vi "TextEditTable.vi"() -> ()   [LabVIEW 2018]
doc: "Handle edits in a text table, limited to column 0\nClick mouse to start edit, Enter to finish edit.\n\n* React to Enter key to complete edit\n* Grab cell one row above the current edit cell (because the table has already responded to the Enter key by moving the current edit cell down by one)\n* Limit edits to only certain rows/cols or cells by changing focus to a dummy offscreen control. (Note: if this dummy control is \"hidden\", this trick won't work).\n* I used a sequence structure to ensure that data gets pulled from table cell _after_ edit has completed (otherwise, it would pull the data before the edit was done)\n*escape key automatically works as it should: it gives up focus and returns the edit cell contents to the string that was there before the edit.\n\nCopyright © 2011 Epimedia, Inc. All Rights Reserved.\n\nThe Epimedia Application Library is Copyright © 2009-2011 Epimedia, Inc. \nAll Rights Reserved. Used under license."
uses:
  <vilib>/Utility/miscctls.llb/LVRowAndColumnTypeDef.ctl
  <vilib>/event_ctls.llb/lveventtype.ctl
  <vilib>/event_ctls.llb/eventvkey.ctl
panel:
  out "SavedDataAfterEdit":string
  in  "DummyButton":bool
  out "Mods":cluster{"Num Pad":bool, "Menu Key":bool}
  out "ScanCode":i16
  out "VKey":T1
  out "Char":i16
  out "Type":T2
  in  "stop":bool
  out "CellValBeforeEdit":string
  out "Active Cell:Active Cell":T3
  in  "Worker Status":string[][](table)
  # "Copyright © 2011 Epimedia, Inc. All Rights Reserved.\n\nThe Epimedia Application Library is Copyright © 2009-2011 Epimedia, Inc. \nAll Rights Reserved. Used under license."
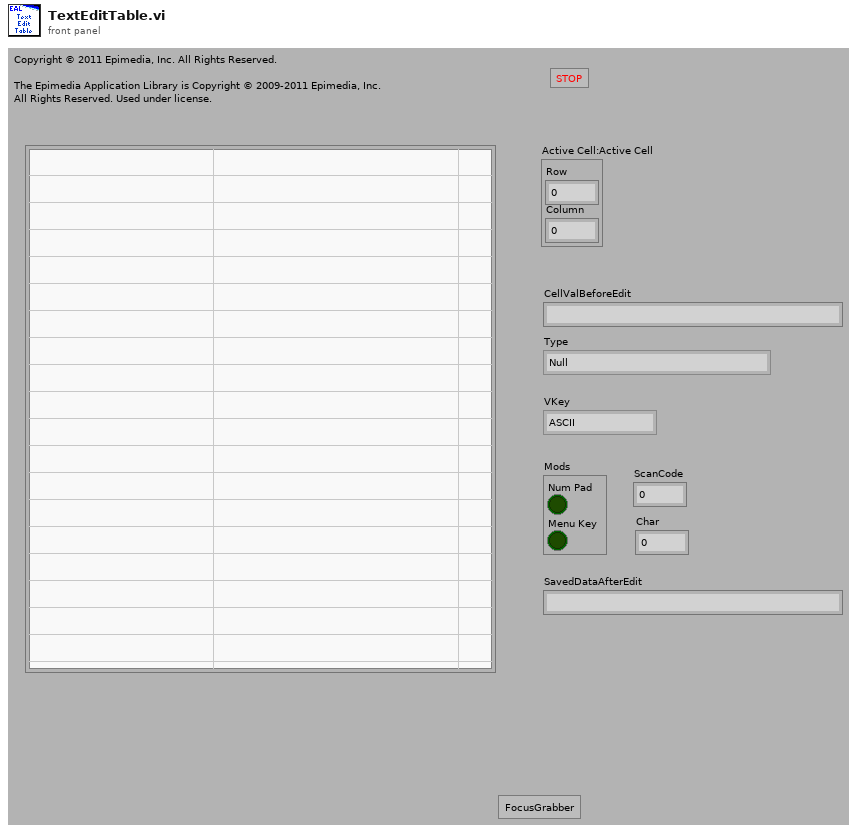
[diagram p1: front panel]
types:
  T1 = typedef "eventvkey.ctl" = enum16{"ASCII", "Enter", "Return", "Shift", "Ctrl", "Alt", "Cmd", "Opt", "Caps", "NumLock", "Clear", "Break", "Up", "Down", "Left", "Right", "Insert", "Delete", "Home", "End", "PageUp", "PageDown", "Escape", "Help", "Pause", "ScrollLock", "F1", "F2", "F3", "F4", "F5", "F6", "F7", "F8", "F9", "F10", "F11", "F12", "F13", "F14", "F15", "F16", "F17", "F18", "F19", "F20", "F21", "F22", "F23", "F24", "Play", "VolumeUp", "VolumeDown", "Mute", "Two Byte Char"}
  T2 = typedef "lveventtype.ctl" = enum32{"Null", "Timeout", "Annotation Menu Selection", "Annotation Menu Selection?", "App Instance Close", "App Instance Close?", "Autoscale Range Change", "Bookmark Info Change", "Cell Edit", "Cell Edit?", "Cursor Grab", "Cursor Grab?", "Cursor Menu Selection", "Cursor Menu Selection?", "Cursor Move", "Cursor Release", "Data Change", "Direction Change", "Display State Change", "Drag Ended", "Drag Enter", "Drag Leave", "Drag Over", "Drag Source Update", "Drag Starting", "Drag Starting?", "Drop", "Exec State Change", "Key Down", "Key Down?", "Key Repeat", "Key Repeat?", "Key Up", "Listbox Double Click", "Menu Activation?", "Menu Selection (App)", "Menu Selection? (App)", "Menu Selection (User)", "Mouse Down", "Mouse Down?", "Mouse Enter", "Mouse Leave", "Mouse Move", "Mouse Up", "Mouse Wheel", "NI Security User Change (App)", "Pane Size", "Panel Close", "Panel Close?", "Panel Resize", "Plot Attribute Change", "Scale Range Change", "Shortcut Menu Activation?", "Shortcut Menu Selection (App)", "Shortcut Menu Selection? (App)", "Shortcut Menu Selection (User)", "Tree Double Click", "Tree Drag", "Tree Drag?", "Tree Drop", "Tree Drop?", "Tree Item Close", "Tree Item Close?", "Tree Item Open", "Tree Item Open?", "User Event", "Value Change"}
  T3 = typedef "LVRowAndColumnTypeDef.ctl" = cluster{"Row":i32, "Column":i32}
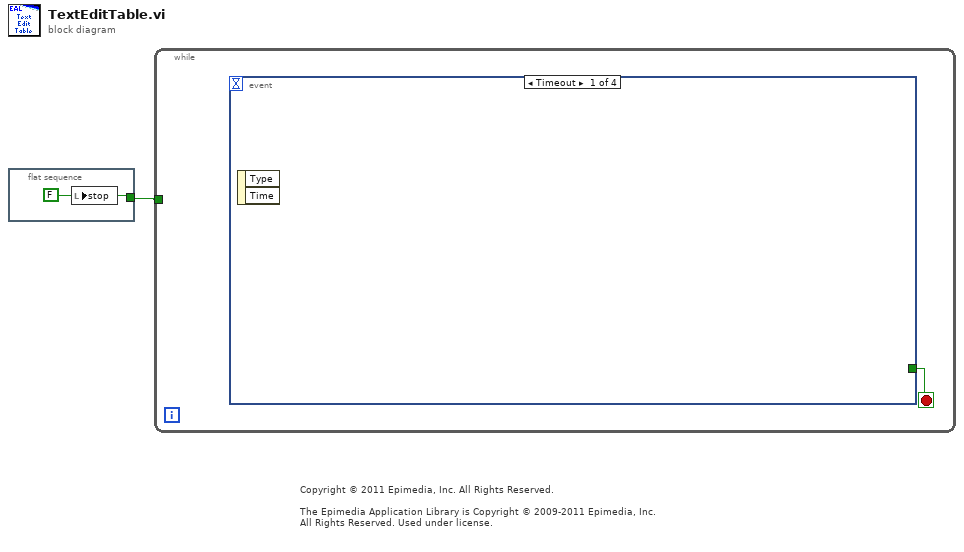
[diagram p0: block diagram]
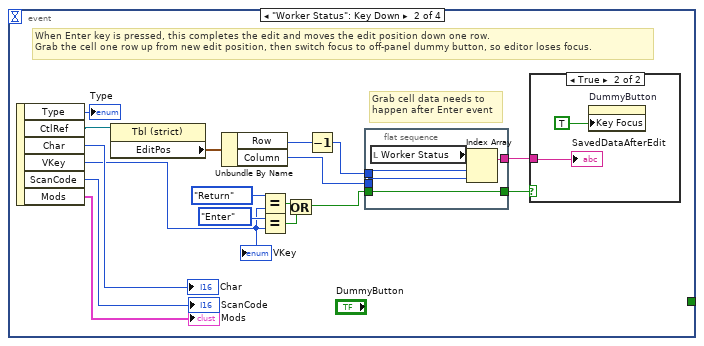
[diagram p2: hidden frame]
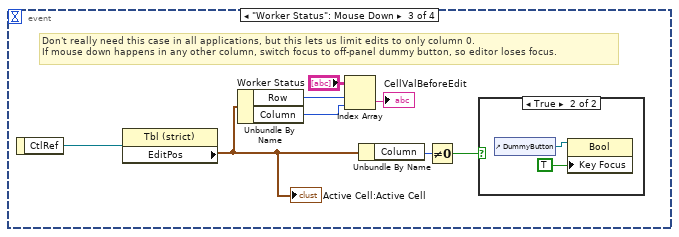
[diagram p4: hidden frame]
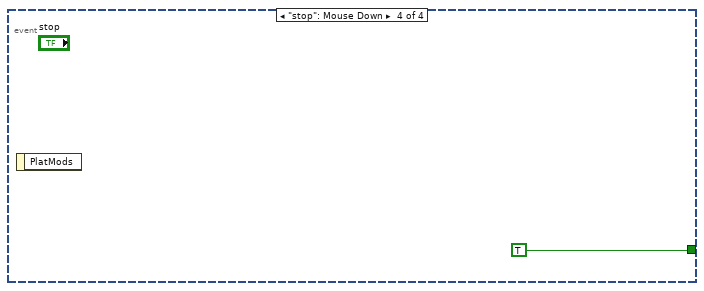
[diagram p6: hidden frame]
diagram:
  # "Copyright © 2011 Epimedia, Inc. All Rights Reserved.\n\nThe Epimedia Application Library is Copyright © 2009-2011 Epimedia, Inc. \nAll Rights Reserved. Used under license."
  n1 = flat-sequence {
    tunnel: [w2] -> w1
    frame #0 {
      w2 = FALSE ("stop")
      n2 = local write "stop"(w2) -> ()
    }
  }
  n3 = while {
    tunnel: w1 -> [_]
    stop <- w3 stop-if-true
    n4 = event shown="[0] Timeout" {
      selector: _ -> [_ _ _ _]
      dyn-events: _ -> [_ _ _ _]
      timeout: _ -> [_ _ _ _]
      tunnel: [_ _ _ TRUE] -> w3
      event Timeout {
        n5 = event-data() -> ()  [unwired: 1 in, 2 out]
      }
      event "Worker Status": Key Down {
        # "Grab cell data needs to \nhappen after Enter event"
        # "When Enter key is pressed, this completes the edit and moves the edit position down one row.\nGrab the cell one row up from new edit position, then switch focus to off-panel dummy button, so editor loses focus."
        n6 = event-data() -> ("Type"=→"Type":T2, "CtlRef"=w19:refnum<vi>, "Char"=→"Char":i16, "VKey"=w9:T1, "ScanCode"=→"ScanCode":i16, "Mods"=→"Mods":cluster{"Num Pad":bool, "Menu Key":bool})  [unwired: 1 in]
        "VKey" <- w9
        n7 = property class="Tbl (strict)"(reference=w19) -> ("EditPos"=w7:T3)  [unwired: 1 in, 2 out]
        n8 = Unbundle By Name(w7) -> ("Row"=w17:i32, "Column"=w18:i32)
        n9 = Equal?(x=eventvkey."Return" ("VKey"), y=w9) -> (x = y?=w13:bool)
        n10 = Equal?(x=eventvkey."Enter" ("VKey"), y=w9) -> (x = y?=w12:bool)
        n11 = Or(x=w13, y=w12) -> (x .or. y?=w5:bool)
        n12 = Decrement(x=w17) -> (x-1=w6:i32)
        n13 = flat-sequence {
          tunnel: w18 -> [w25]
          tunnel: [w23] -> w8
          tunnel: w6 -> [w22]
          tunnel: w5 -> [w21]
          tunnel: [w21] -> w4
          frame #0 {
            n14 = local read "Worker Status"() -> (w24:string[][])
            n15 = Index Array(array=w24, index (row)=w22, index (col)=w25) -> (element=w23:string)
          }
        }
        n16 = case shown="True" w4 {
          tunnel: w8 -> [_ w26]
          frame False {
          }
          frame True {
            n17 = property on="DummyButton" class="Bool"("Key Focus"=TRUE) -> ()  [unwired: 2 in, 2 out]
            "SavedDataAfterEdit" <- w26
          }
        }
      }
      event "Worker Status": Mouse Down {
        # "Don't really need this case in all applications, but this lets us limit edits to only column 0. \nIf mouse down happens in any other column, switch focus to off-panel dummy button, so editor loses focus."
        n18 = event-data() -> ("CtlRef"=w35:refnum<vi>)  [unwired: 1 in]
        n19 = property class="Tbl (strict)"(reference=w35) -> ("EditPos"=w30:T3)  [unwired: 1 in, 2 out]
        "Active Cell:Active Cell" <- w30
        n20 = Unbundle By Name(w30) -> ("Row"=w34:i32, "Column"=w32:i32)
        n21 = Index Array(array="Worker Status", index (row)=w34, index (col)=w32) -> (element=→"CellValBeforeEdit":string)
        n22 = Unbundle By Name(w30) -> ("Column"=w28:i32)
        n23 = Not Equal To 0?(x=w28) -> (x != 0?=w29:bool)
        n24 = case shown="True" w29 {
          frame False {
          }
          frame True {
            n25 = control-ref of="DummyButton"() -> (w36:refnum<vi>)
            n26 = property on="Property Node" class="Bool"(reference=w36, "Key Focus"=TRUE) -> ()  [unwired: 1 in, 2 out]
          }
        }
      }
      event "stop": Mouse Down {
        n27 = event-data() -> ()  [unwired: 1 in, 1 out]
      }
    }
  }
